vi "GetLastSavedVbreak.vi"(0 "storage refnum (file)":refnum<k20>, 1 "error in":errorcluster) -> (2 "storage refnum (file) out":refnum<k20>, 3 "VBreak":dbl, 4 "error out":errorcluster)   [LabVIEW 2014]
uses:
  <vilib>/Platform/storage/lvStorage.llb/_queryPropPoly.vi
  <vilib>/Platform/storage/lvStorage.llb/_queryPropString.vi
  <vilib>/Platform/storage/lvStorage.llb/_queryGenericObjects.vi
  <vilib>/Platform/storage/lvStorage.llb/_loadAllDdt.vi
  <vilib>/Platform/storage/lvStorage.llb/xStorage/xStorageSupp/ErrorOut.vi
  <vilib>/Platform/storage/lvStorage.llb/xStorage/Read Data/Read Data.xnode
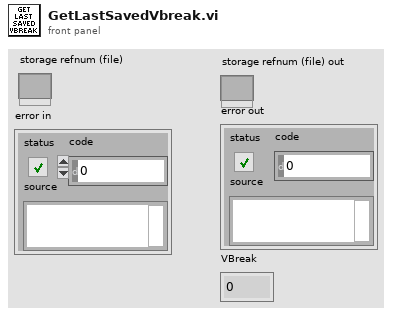
[diagram p1: front panel]
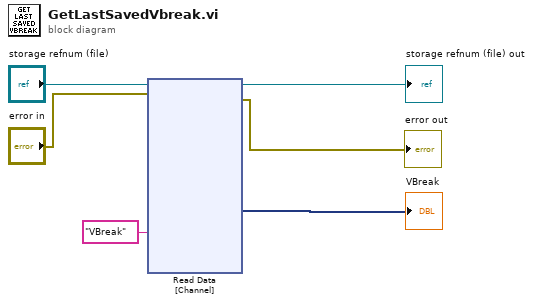
[diagram p0: block diagram]
diagram:
  n1 = xnode "Read Data\n[Channel]"("Name"="VBreak", "storage refnum (file)"="storage refnum (file)", "error in"="error in") -> ("Signal"=→"VBreak":dynamicdata, "storage refnum (file) out"=→"storage refnum (file) out":refnum<k20>, "error out"=→"error out":errorcluster)  [unwired: 3 in, 1 out]
